vi "ExSubCreateImageAdjSizeDisplay.vi"(0 "Camera Handle":u32=16842752, 1 "Pulser Handle":u32, 2 "File and Display Name":string="test", 3 "error in (no error)":errorcluster, 4 "divider":i32=1) -> (5 "Handles Out":T1={"Camera Handle"=16842752, "Pulser Handle"=0, "File Handle"=0, "Display Handle"=0, "Image Handle"=1}, 7 "error out":errorcluster)   [LabVIEW 2010]
panel:
  # "ExSubCreateFileMultImage.vi:\nThis is a SubVI that creates a file,  and image objects and returns the handles bundled in a cluster that includes a pulser and camera handle"
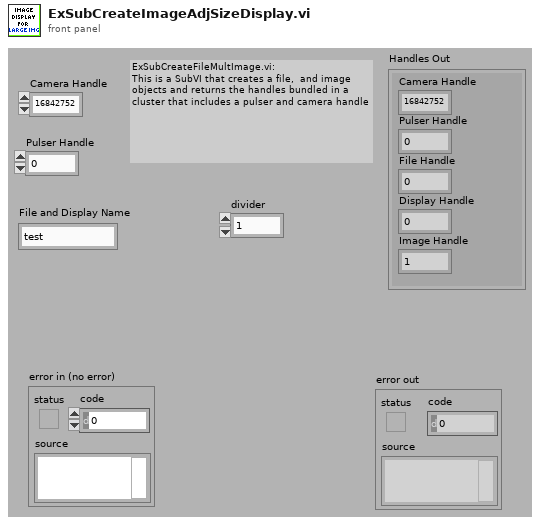
[diagram p1: front panel]
types:
  T1 = cluster{"Camera Handle":u32, "Pulser Handle":u32, "File Handle":u32, "Display Handle":u32, "Image Handle":u32}
  T2 = cluster{"Camera Handle":u32, "Pulser Handle":u32, i32, "Display Handle":u32, "Image Handle":u32}
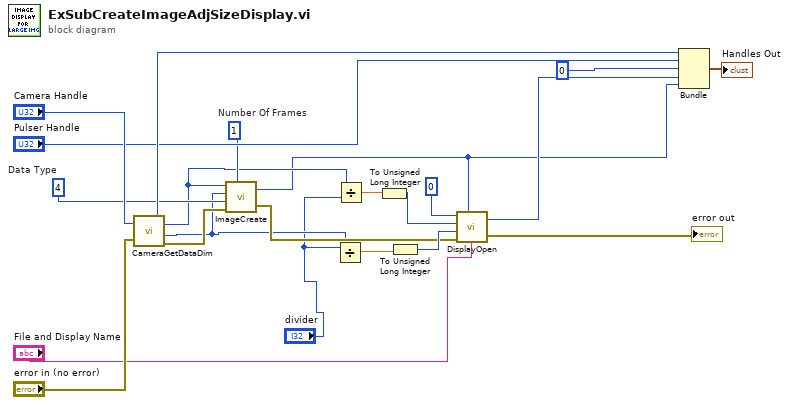
[diagram p0: block diagram]
diagram:
  w7 = u32 4  # Data Type
  w8 = u32 1  # Number Of Frames
  n1 = call <userlib>:"CameraGetDataDim.vi"("Camera Handle"="Camera Handle", "error in"="error in (no error)") -> ("Camera Handle"=w20:u32, "Xdim"=w6:u32, "Ydim"=w5:u32, "error out"=w10:errorcluster)
  n2 = call <userlib>:"ImageCreate.vi"("X dimension"=w6, "Y dimension"=w5, "Data Type"=w7, "error in"=w10, "Number Of Frames"=w8) -> ("Image Handle"=w2:u32, "error out"=w9:errorcluster)
  n3 = Divide(x=w5, y="divider") -> (x/y=w15:dbl)
  n4 = Divide(x=w6, y="divider") -> (x/y=w13:dbl)
  n5 = To Unsigned Long Integer(number=w13) -> (unsigned 32bit integer=w12:u32)
  n6 = To Unsigned Long Integer(number=w15) -> (unsigned 32bit integer=w14:u32)
  n7 = call <userlib>:"DisplayOpen.vi"("Display Title"="File and Display Name", "Image Handle"=w2, "error in"=w9, "Display Height"=w14, "Display Width"=w12, "Display Type"=0) -> ("error out"=→"error out":errorcluster, "Display Handle"=w18:u32)
  n8 = Bundle("Camera Handle"=w20, "Pulser Handle"="Pulser Handle", 0, "Display Handle"=w18, "Image Handle"=w2) -> (→"Handles Out":T2)  [unwired: 1 in]
